vi "Main.vi"() -> ()   [LabVIEW 2023]
doc: "This Continuous Measurement sample project is based on the Queued Message Handler template.\n\nThe Event Handling Loop generates messages based on user interface actions.\n\nThe Message Handling Loop processes messages generated by the Event Handling Loop, or by other messages. There are also Acquisition and Logging message handling loop subVIs, and a chart updating loop."
uses:
  controls/UI Data.ctl
  controls/UI State.ctl
  support/Message Queue/Enqueue Message (Single).vi
  <vilib>/Utility/error.llb/Error Cluster From Error Code.vi
  <vilib>/ErrorRing/Error Ring.xnode
  Acquisition/Acquisition.lvlib
  Logging/Logging.lvlib
  support/User Event - Stop/User Event - Stop.lvlib
  support/Message Queue/Message Queue.lvlib
panel:
  out "CPU":dbl
  out "Data":u32(graph)
  in  "Start":bool
  in  "Stop":bool
  out "Status":string
  in  "Exit":bool
  # "Continuous Measurement Data Logger"
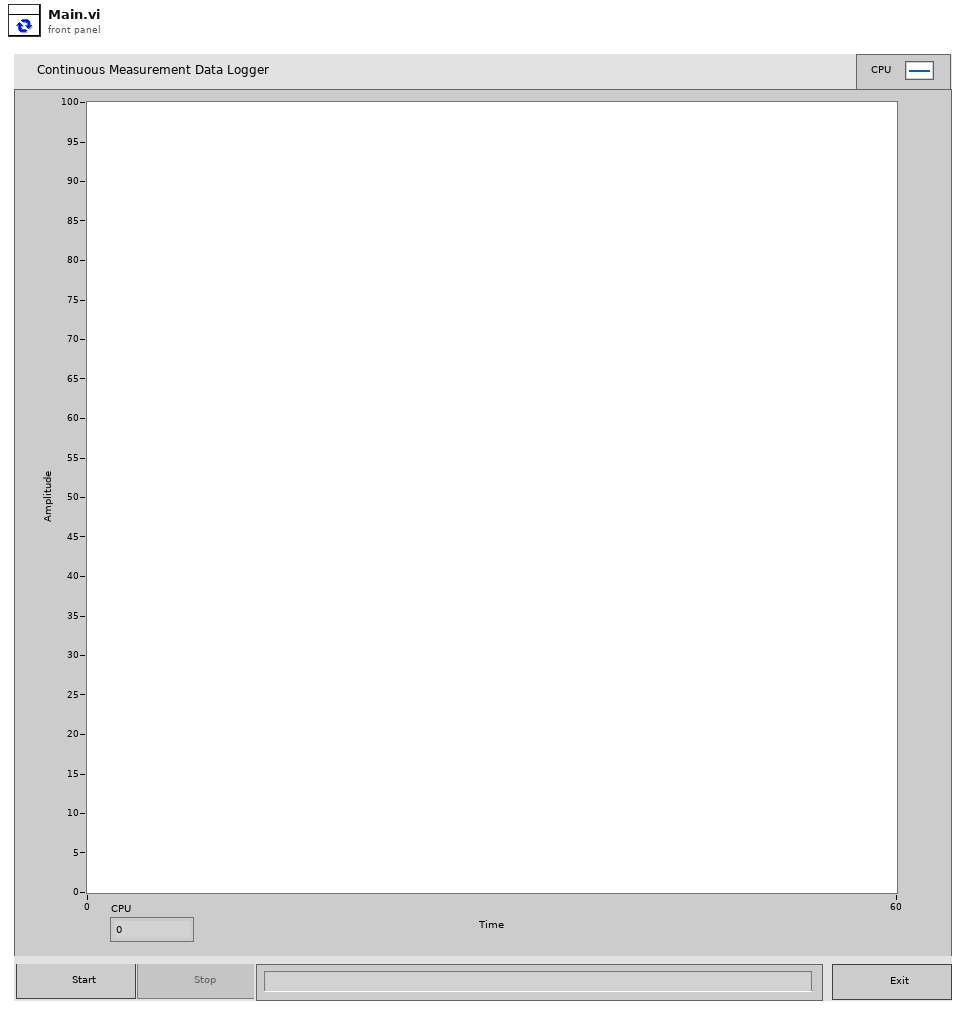
[diagram p1: front panel]
types:
  T1 = typedef "UI State.ctl" = enum16{"Idle", "Acquiring and Logging", "Waiting for Exit", "Waiting for Exit (Acq Stopped)", "Waiting for Exit (Log Stopped)", "Waiting for Stop", "Waiting for Stop (Acq Stopped)", "Waiting for Stop (Log Stopped)"}
  T2 = typedef "UI Data.ctl" = cluster{"Start Ref":refnum<vi>, "Stop Ref":refnum<vi>, "Settings Ref":refnum<vi>, "Exit Ref":refnum<vi>, "Status Ref":refnum<vi>, "Data Ref":refnum<vi>}
  T3 = typedef "Message Queue.lvlib/All Message Queues.ctl" = cluster{"UI":refnum<queue>, "Acquisition":refnum<queue>, "Logging":refnum<queue>}
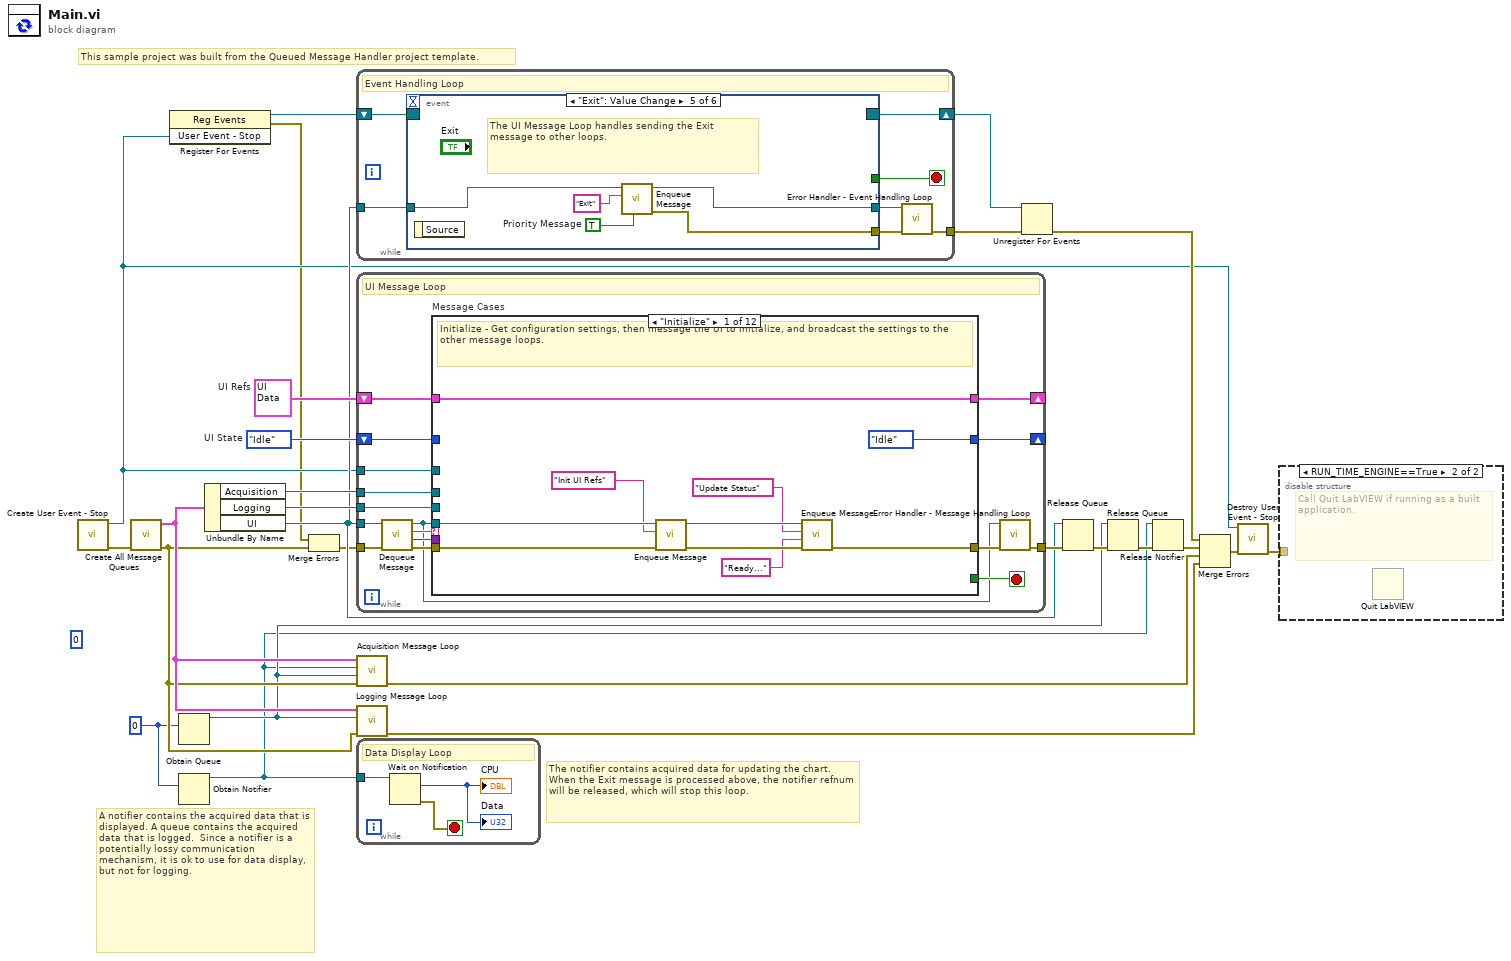
[diagram p0: block diagram]
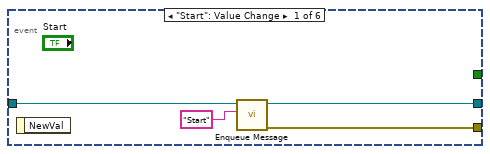
[diagram p3: hidden frame]
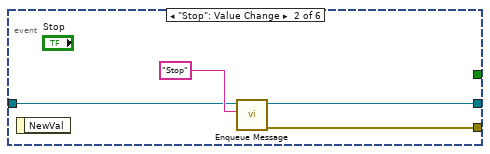
[diagram p4: hidden frame]
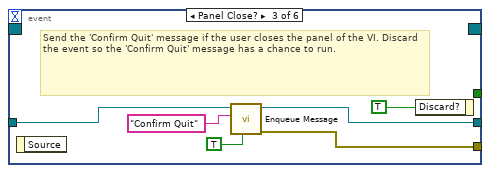
[diagram p5: hidden frame]
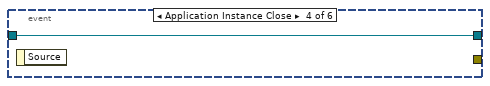
[diagram p6: hidden frame]
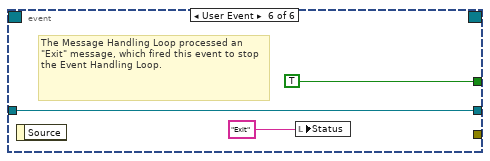
[diagram p7: hidden frame]
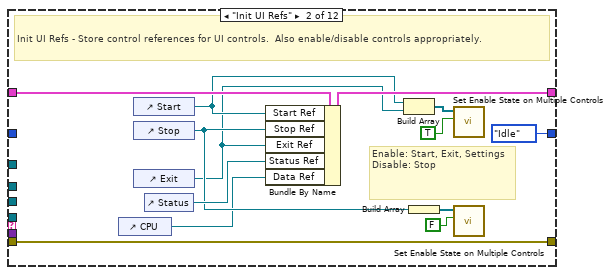
[diagram p8: hidden frame]
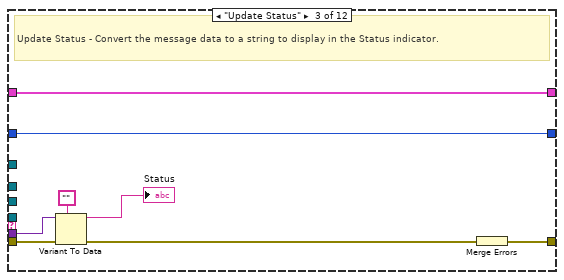
[diagram p9: hidden frame]
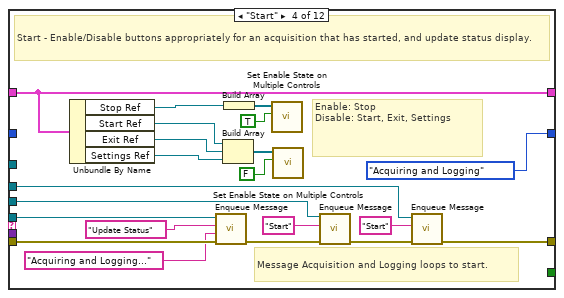
[diagram p10: hidden frame]
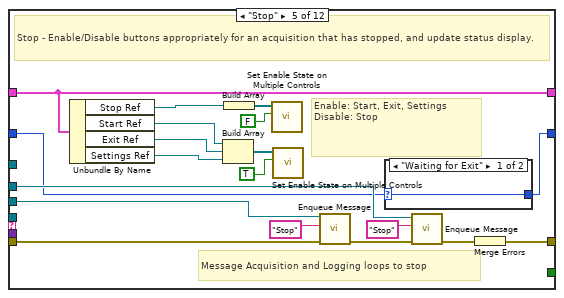
[diagram p11: hidden frame]
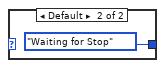
[diagram p12: hidden frame]
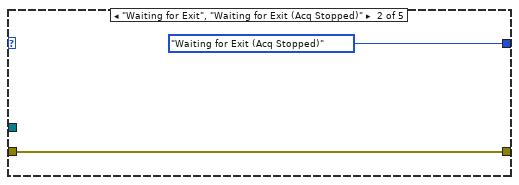
[diagram p14: hidden frame]
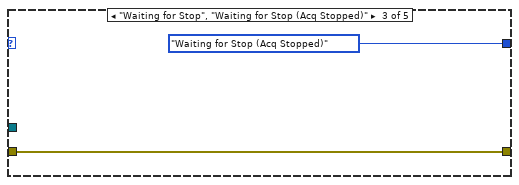
[diagram p15: hidden frame]
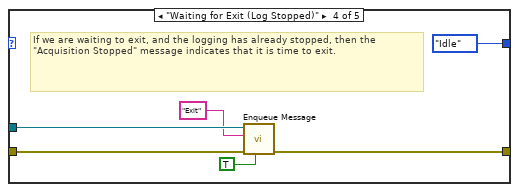
[diagram p16: hidden frame]
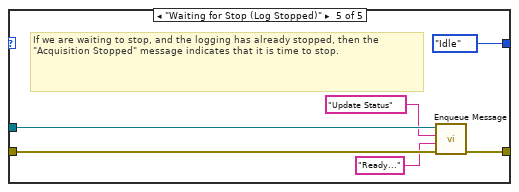
[diagram p17: hidden frame]
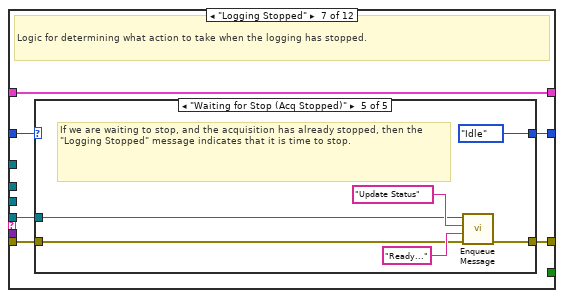
[diagram p18: hidden frame]
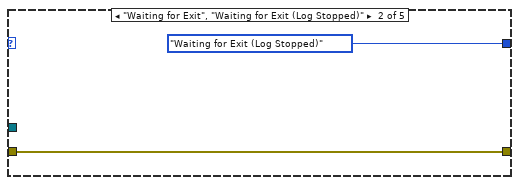
[diagram p20: hidden frame]
diagram:
  (unwired) u32 0 ("notification")
  w1 = u32 0 ("CPU load 2")
  w14 = UI_State."Idle"  # UI State
  w17 = T2 {"Start Ref"=refnum, "Stop Ref"=refnum, "Settings Ref"=refnum, "Exit Ref"=refnum, "Status Ref"=refnum, "Data Ref"=refnum}  # UI Refs
  # "This sample project was built from the Queued Message Handler project template."
  # "A notifier contains the acquired data that is displayed. A queue contains the acquired data that is logged.  Since a notifier is a potentially lossy communication mechanism, it is ok to use for data display, but not for logging."
  # "The notifier contains acquired data for updating the chart. When the Exit message is processed above, the notifier refnum will be released, which will stop this loop."
  n1 = call "Create User Event - Stop.vi"() -> ("error out"=w23:errorcluster, "User Event - Stop"=w4:refnum<user-event>)  [unwired: 10 in]
  n2 = call "Create All Message Queues.vi"("error in (no error)"=w23) -> ("error out"=w20:errorcluster, "Message Queues out"=w22:T3)  [unwired: 9 in]
  n3 = register-events(w4) -> (reference out=w5:refnum<event-registration>, error out=w2:errorcluster)  [unwired: 2 in]
  n4 = Obtain Queue(element data type=w1) -> (queue out=w7:refnum<queue>)  [unwired: 4 in, 2 out]
  n5 = Obtain Notifier(notification data type=w1) -> (notifier out=w6:refnum<notifier>)  [unwired: 3 in, 2 out]
  n6 = Unbundle By Name(w22) -> ("Acquisition"=w16:refnum<queue>, "Logging"=w15:refnum<queue>, "UI"=w12:refnum<queue>)
  n7 = Merge Errors(w2, w20) -> (w3:errorcluster)
  n8 = while {
    tunnel: w12 -> [w32]
    tunnel: [w29] -> w25
    shift-right: [w31] -> w18
    shift-left: w5 -> [w33]
    stop <- w30 stop-if-true
    # "Event Handling Loop"
    n9 = event shown="[4] \"Exit\": Value Change" {
      selector: w33 -> [_ _ _ _ _ _]
      dyn-events: [_ _ _ _ _ _] -> w31
      timeout: _ -> [_ _ _ _ _ _]
      tunnel: [_ _ _ _ _ TRUE ("Discard?")] -> w30
      tunnel: w32 -> [w37 w40 w45 w48 w50 w54]
      tunnel: [w35 w39 w43 _ w53 _] -> w28
      tunnel: [w34 w38 w44 w48 w49 w54] -> w27
      event "Start": Value Change {
        n10 = event-data() -> ()  [unwired: 1 in, 1 out]
        n11 = call-poly "Enqueue Message.vi"("Message"="Start", "Message Queue"=w37) -> ("error out"=w35:errorcluster, "dup Message Queue"=w34:refnum<queue>)  [unwired: 8 in]
      }
      event "Stop": Value Change {
        n12 = event-data() -> ()  [unwired: 1 in, 1 out]
        n13 = call-poly "Enqueue Message.vi"("Message"="Stop", "Message Queue"=w40) -> ("error out"=w39:errorcluster, "dup Message Queue"=w38:refnum<queue>)  [unwired: 8 in]
      }
      event Panel Close? {
        # "Send the 'Confirm Quit' message if the user closes the panel of the VI. Discard the event so the 'Confirm Quit' message has a chance to run."
        n14 = event-data() -> ()  [unwired: 1 in, 1 out]
        n15 = call-poly "Enqueue Message.vi"("Priority Message? (F)"=TRUE, "Message"="Confirm Quit", "Message Queue"=w45) -> ("error out"=w43:errorcluster, "dup Message Queue"=w44:refnum<queue>)  [unwired: 7 in]
        n16 = event-data("Discard?"=TRUE) -> ()  [unwired: 1 in, 1 out]
      }
      event Application Instance Close {
        n17 = event-data() -> ()  [unwired: 1 in, 1 out]
      }
      event "Exit": Value Change {
        w51 = TRUE  # Priority Message
        # "The UI Message Loop handles sending the Exit message to other loops."
        n18 = event-data() -> ()  [unwired: 1 in, 1 out]
        n19 = call-poly "Enqueue Message.vi"("Priority Message? (F)"=w51, "Message"="Exit", "Message Queue"=w50) -> ("error out"=w53:errorcluster, "dup Message Queue"=w49:refnum<queue>)  [unwired: 7 in]
      }
      event User Event {
        # "The Message Handling Loop processed an \"Exit\" message, which fired this event to stop the Event Handling Loop."
        n20 = event-data() -> ()  [unwired: 1 in, 1 out]
        n21 = local write "Status"("Exit" ("Exit String")) -> ()
      }
    }
    n22 = call "Error Handler - Event Handling Loop.vi"("error in (no error)"=w28, "Message Queue"=w27) -> ("dup error in"=w29:errorcluster)  [unwired: 8 in, 1 out]
  }
  n23 = while {
    tunnel: w12 -> [w66]
    tunnel: w4 -> [w71]
    shift-right: [w64] -> _
    shift-left: w17 -> [w65]
    tunnel: w16 -> [w63]
    tunnel: w15 -> [w62]
    shift-right: [w57] -> _
    shift-left: w14 -> [w58]
    tunnel: w3 -> [w70]
    tunnel: [w61] -> w26
    stop <- w72 stop-if-true
    # "UI Message Loop"
    n24 = call "Dequeue Message.vi"("error in (no error)"=w70, "Message Queue"=w66) -> ("error out"=w69:errorcluster, "Message Data"=w67:variant, "Message"=w68:string, "dup Message Queue"=w59:refnum<queue>)  [unwired: 6 in]
    n25 = case "Message Cases" shown="\"Initialize\"" w68 {
      selector: w68 -> [_ _ _ _ _ _ _ _ _ _ _ w249]
      tunnel: w59 -> [w76 _ _ w124 _ w148 w172 _ w205 _ _ _]
      tunnel: w69 -> [w75 w95 w102 w123 w142 w149 w173 w194 w204 w232 w247 _]
      tunnel: [w80 w95 w103 w107 w143 w146 w170 w197 w203 w241 w246 w248] -> w60
      tunnel: [_ _ _ _ _ _ _ _ _ TRUE _ _] -> w72
      tunnel: w67 -> [_ _ w101 _ _ _ _ w198 _ w230 _ _]
      tunnel: w71 -> [_ _ _ _ _ _ _ _ _ w242 _ _]
      tunnel: w65 -> [w77 w94 w97 w120 w141 w151 w175 w201 w207 w240 w245 w251]
      tunnel: [w77 w92 w97 w120 w141 w151 w175 w201 w207 w240 w245 w251] -> w64
      tunnel: w63 -> [_ _ _ w106 w128 _ _ _ _ w239 _ _]
      tunnel: w62 -> [_ _ _ w109 w131 _ _ _ _ w238 _ _]
      tunnel: w58 -> [_ _ w96 _ w125 w150 w174 w196 w206 _ w244 w250]
      tunnel: [UI_State."Idle" ("UI State") UI_State."Idle" ("UI State") w96 UI_State."Acquiring and Logging" ("UI State") w126 w147 w171 w196 w202 UI_State."Idle" ("UI State") w244 w250] -> w57
      frame "Initialize" {
        # "Initialize - Get configuration settings, then message the UI to initialize, and broadcast the settings to the other message loops."
        n26 = call-poly "Enqueue Message.vi"("error in (no error)"=w75, "Message"="Init UI Refs", "Message Queue"=w76) -> ("error out"=w82:errorcluster, "dup Message Queue"=w81:refnum<queue>)  [unwired: 7 in]
        n27 = call-poly "Enqueue Message.vi"("error in (no error)"=w82, "Message Data"="Ready..." ("Ready..."), "Message"="Update Status", "Message Queue"=w81) -> ("error out"=w80:errorcluster)  [unwired: 6 in, 1 out]
      }
      frame "Init UI Refs" {
        # "Enable: Start, Exit, Settings\nDisable: Stop"
        # "Init UI Refs - Store control references for UI controls.  Also enable/disable controls appropriately."
        n28 = control-ref of="CPU"() -> (w83:refnum<vi>)
        n29 = control-ref of="Start"() -> (w86:refnum<vi>)
        n30 = control-ref of="Stop"() -> (w87:refnum<vi>)
        n31 = control-ref of="Exit"() -> (w84:refnum<vi>)
        n32 = control-ref of="Status"() -> (w93:refnum<vi>)
        n33 = Bundle By Name(cluster=w94, "Start Ref"=w86, "Stop Ref"=w87, "Exit Ref"=w84, "Status Ref"=w93, "Data Ref"=w83) -> (w92:T2)
        n34 = Build Array(w86, w84) -> (w90:refnum<vi>[])
        n35 = Build Array(w87) -> (w89:refnum<vi>[])
        n36 = call "Set Enable State on Multiple Controls.vi"("Enable?"=TRUE, "Controls"=w90) -> ()  [unwired: 10 in]
        n37 = call "Set Enable State on Multiple Controls.vi"("Enable?"=FALSE, "Controls"=w89) -> ()  [unwired: 10 in]
      }
      frame "Update Status" {
        # "Update Status - Convert the message data to a string to display in the Status indicator."
        n38 = Variant To Data(error in=w102, type="", Variant=w101) -> (data=→"Status":string, error out=w99:errorcluster)
        n39 = Merge Errors(w99) -> (w103:errorcluster)
      }
      frame "Start" {
        # "Message Acquisition and Logging loops to start."
        # "Enable: Stop\nDisable: Start, Exit, Settings"
        # "Start - Enable/Disable buttons appropriately for an acquisition that has started, and update status display."
        n40 = Unbundle By Name(w120) -> ("Stop Ref"=w115:refnum<vi>, "Start Ref"=w114:refnum<vi>, "Exit Ref"=w113:refnum<vi>, "Settings Ref"=w112:refnum<vi>)
        n41 = call-poly "Enqueue Message.vi"("error in (no error)"=w123, "Message Data"="Acquiring and Logging..." ("Acquiring and Logging..."), "Message"="Update Status", "Message Queue"=w124) -> ("error out"=w111:errorcluster)  [unwired: 6 in, 1 out]
        n42 = Build Array(w114, w113, w112) -> (w118:refnum<vi>[])
        n43 = Build Array(w115) -> (w117:refnum<vi>[])
        n44 = call "Set Enable State on Multiple Controls.vi"("Enable?"=TRUE, "Controls"=w117) -> ()  [unwired: 10 in]
        n45 = call "Set Enable State on Multiple Controls.vi"("Enable?"=FALSE, "Controls"=w118) -> ()  [unwired: 10 in]
        n46 = call-poly "Enqueue Message.vi"("error in (no error)"=w111, "Message"="Start", "Message Queue"=w109) -> ("error out"=w108:errorcluster)  [unwired: 7 in, 1 out]
        n47 = call-poly "Enqueue Message.vi"("error in (no error)"=w108, "Message"="Start", "Message Queue"=w106) -> ("error out"=w107:errorcluster)  [unwired: 7 in, 1 out]
      }
      frame "Stop" {
        # "Message Acquisition and Logging loops to stop"
        # "Enable: Start, Exit, Settings\nDisable: Stop"
        # "Stop - Enable/Disable buttons appropriately for an acquisition that has stopped, and update status display."
        n48 = Unbundle By Name(w141) -> ("Stop Ref"=w136:refnum<vi>, "Start Ref"=w135:refnum<vi>, "Exit Ref"=w134:refnum<vi>, "Settings Ref"=w133:refnum<vi>)
        n49 = Build Array(w135, w134, w133) -> (w139:refnum<vi>[])
        n50 = Build Array(w136) -> (w138:refnum<vi>[])
        n51 = call "Set Enable State on Multiple Controls.vi"("Enable?"=FALSE, "Controls"=w138) -> ()  [unwired: 10 in]
        n52 = call "Set Enable State on Multiple Controls.vi"("Enable?"=TRUE, "Controls"=w139) -> ()  [unwired: 10 in]
        n53 = call-poly "Enqueue Message.vi"("error in (no error)"=w142, "Message"="Stop", "Message Queue"=w131) -> ("error out"=w130:errorcluster)  [unwired: 7 in, 1 out]
        n54 = case shown="\"Waiting for Exit\"" w125 {
          selector: w125 -> [w144 _]
          tunnel: [w144 UI_State."Waiting for Stop" ("UI State")] -> w126
          frame "Waiting for Exit" {
          }
          frame Default {
          }
        }
        n55 = call-poly "Enqueue Message.vi"("error in (no error)"=w130, "Message"="Stop", "Message Queue"=w128) -> ("error out"=w129:errorcluster)  [unwired: 7 in, 1 out]
        n56 = Merge Errors(w129) -> (w143:errorcluster)
      }
      frame "Acquisition Stopped" {
        # "Logic for determining what action to take when the acquisition has stopped."
        n57 = case shown="Default" w150 {
          selector: w150 -> [w153 _ _ _ _]
          tunnel: w149 -> [w152 w155 w157 w163 w169]
          tunnel: w148 -> [_ _ _ w161 w166]
          tunnel: [w153 UI_State."Waiting for Exit (Acq Stopped)" ("UI State") UI_State."Waiting for Stop (Acq Stopped)" ("UI State") UI_State."Idle" ("UI State") UI_State."Idle" ("UI State")] -> w147
          tunnel: [w152 w155 w157 w162 w167] -> w146
          frame Default {
          }
          frame "Waiting for Exit", "Waiting for Exit (Acq Stopped)" {
          }
          frame "Waiting for Stop", "Waiting for Stop (Acq Stopped)" {
          }
          frame "Waiting for Exit (Log Stopped)" {
            # "If we are waiting to exit, and the logging has already stopped, then the \"Acquisition Stopped\" message indicates that it is time to exit."
            n58 = call-poly "Enqueue Message.vi"("Priority Message? (F)"=TRUE, "error in (no error)"=w163, "Message"="Exit", "Message Queue"=w161) -> ("error out"=w162:errorcluster)  [unwired: 6 in, 1 out]
          }
          frame "Waiting for Stop (Log Stopped)" {
            # "If we are waiting to stop, and the logging has already stopped, then the \"Acquisition Stopped\" message indicates that it is time to stop."
            n59 = call-poly "Enqueue Message.vi"("error in (no error)"=w169, "Message Data"="Ready..." ("Ready..."), "Message"="Update Status", "Message Queue"=w166) -> ("error out"=w167:errorcluster)  [unwired: 6 in, 1 out]
          }
        }
      }
      frame "Logging Stopped" {
        # "Logic for determining what action to take when the logging has stopped."
        n60 = case shown="\"Waiting for Stop (Acq Stopped)\"" w174 {
          selector: w174 -> [w177 _ _ _ _]
          tunnel: w173 -> [w176 w179 w181 w187 w190]
          tunnel: w172 -> [_ _ _ w185 w189]
          tunnel: [w177 UI_State."Waiting for Exit (Log Stopped)" ("UI State") UI_State."Waiting for Stop (Log Stopped)" ("UI State") UI_State."Idle" ("UI State") UI_State."Idle" ("UI State")] -> w171
          tunnel: [w176 w179 w181 w186 w188] -> w170
          frame Default {
          }
          frame "Waiting for Exit", "Waiting for Exit (Log Stopped)" {
          }
          frame "Waiting for Stop", "Waiting for Stop (Log Stopped)" {
          }
          frame "Waiting for Exit (Acq Stopped)" {
            # "If we are waiting to exit, and the acquisition has already stopped, then the \"Logging Stopped\" message indicates that it is time to exit."
            n61 = call-poly "Enqueue Message.vi"("Priority Message? (F)"=TRUE, "error in (no error)"=w187, "Message"="Exit", "Message Queue"=w185) -> ("error out"=w186:errorcluster)  [unwired: 6 in, 1 out]
          }
          frame "Waiting for Stop (Acq Stopped)" {
            # "If we are waiting to stop, and the acquisition has already stopped, then the \"Logging Stopped\" message indicates that it is time to stop."
            n62 = call-poly "Enqueue Message.vi"("error in (no error)"=w190, "Message Data"="Ready..." ("Ready..."), "Message"="Update Status", "Message Queue"=w189) -> ("error out"=w188:errorcluster)  [unwired: 6 in, 1 out]
          }
        }
      }
      frame "Error" {
        # "Error - Display an error dialog. This message is sent by the \"Error Handler\" VIs at the end of other loops in this application."
        n63 = Variant To Data(error in=w194, type=errorcluster {"status"=FALSE, "code"=0, "source"=""} ("error constant"), Variant=w198) -> (data=w195:errorcluster, error out=w199:errorcluster)
        n64 = call <vilib>:"Simple Error Handler.vi"("error in (no error)"=w195) -> ()  [unwired: 4 in, 5 out]
        n65 = Merge Errors(w199) -> (w197:errorcluster)
      }
      frame "Confirm Quit" {
        # "Confirm Quit - Message that can confirm whether or not the user wants to exit the application."
        n66 = case shown="\"Acquiring and Logging\"" w206 {
          tunnel: w205 -> [w213 w217]
          tunnel: w204 -> [w212 w216]
          tunnel: [w211 w215] -> w203
          tunnel: [UI_State."Idle" ("UI State") w214] -> w202
          frame Default {
            # "If 'Confirm Quit' comes in while the system is idle, there is no need for a confirmation message."
            n67 = call-poly "Enqueue Message.vi"("Priority Message? (F)"=TRUE, "error in (no error)"=w212, "Message"="Exit", "Message Queue"=w213) -> ("error out"=w211:errorcluster)  [unwired: 6 in, 1 out]
          }
          frame "Acquiring and Logging" {
            n68 = Two Button Dialog(message="Are you sure you want to quit while the acquisition is running?" ("Confirm Quit Message"), 1:"No" ("No"), 2:"Yes" ("Yes")) -> (T button?=w218:bool)
            n69 = case shown="True" w218 {
              tunnel: w217 -> [_ w227]
              tunnel: w216 -> [w223 w228]
              tunnel: [w223 w226] -> w215
              tunnel: [UI_State."Acquiring and Logging" ("UI State") UI_State."Waiting for Exit" ("UI State")] -> w214
              frame False {
                # "User did not want to quit."
              }
              frame True {
                n70 = call-poly "Enqueue Message.vi"("error in (no error)"=w228, "Message"="Stop", "Message Queue"=w227) -> ("error out"=w226:errorcluster)  [unwired: 7 in, 1 out]
              }
            }
          }
        }
      }
      frame "Exit" {
        w234 = TRUE ("Priority Message? (F)")
        w235 = "Exit" ("Message")
        # "Popup an error dialog if 'Exit' was called as a result of an error."
        # "Stop the VI"
        # "Exit - Send Exit messages to the Acquisition and Logging loops, and fire the user event to stop the Event Handling Loop."
        n71 = Variant To Data(type=errorcluster {"status"=FALSE, "code"=0, "source"=""} ("error constant"), Variant=w230) -> (data=w229:errorcluster)  [unwired: 1 in, 1 out]
        n72 = call <vilib>:"Simple Error Handler.vi"("error in (no error)"=w229) -> ()  [unwired: 4 in, 5 out]
        n73 = call-poly "Enqueue Message.vi"("Priority Message? (F)"=w234, "error in (no error)"=w232, "Message"=w235, "Message Queue"=w239) -> ("error out"=w236:errorcluster)  [unwired: 6 in, 1 out]
        n74 = call-poly "Enqueue Message.vi"("Priority Message? (F)"=w234, "error in (no error)"=w236, "Message"=w235, "Message Queue"=w238) -> ("error out"=w233:errorcluster)  [unwired: 6 in, 1 out]
        n75 = call "Fire User Event - Stop.vi"("error in (no error)"=w233, "User Event - Stop"=w242) -> ("error out"=w241:errorcluster)  [unwired: 9 in]
      }
      frame "---Copy This Frame---" {
        # "Duplicate this frame when creating new messages.  Change this comment in the duplicated frame to describe this message."
        n76 = Merge Errors(w247) -> (w246:errorcluster)
      }
      frame Default {
        # "'Default' case only runs if there is a message that isn't defined in any of the other cases.  Output a programming error."
        n77 = xnode "Error Ring"("parameter 0"=w249) -> ("error out"=w248:errorcluster)
      }
    }
    n78 = call "Error Handler - Message Handling Loop.vi"("error in (no error)"=w60, "Message Queue"=w59) -> ("dup error in"=w61:errorcluster)  [unwired: 8 in, 1 out]
  }
  n79 = call "Acquisition Message Loop.vi"("error in (no error)"=w20, "Data Queue"=w7, "Data Notifier"=w6, "Message Queues"=w22) -> ("error out"=w24:errorcluster)  [unwired: 7 in]
  n80 = call "Logging Message Loop.vi"("error in (no error)"=w20, "Data Queue"=w7, "Message Queues"=w22) -> ("error out"=w21:errorcluster)  [unwired: 8 in]
  n81 = while "Data Display Loop" {
    tunnel: w6 -> [w261]
    stop <- w260 stop-if-true
    # "Data Display Loop"
    n82 = Wait on Notification(notifier=w261) -> (notification=→"Data" →"CPU":u32, error out=w260:errorcluster)  [unwired: 3 in, 2 out]
  }
  n83 = Unregister For Events(event registration refnum=w18, error in=w25) -> (error out=w19:errorcluster)
  n84 = Release Queue(queue=w12, error in (no error)=w26) -> (error out=w10:errorcluster)  [unwired: 1 in, 2 out]
  n85 = Release Queue(queue=w7, error in (no error)=w10) -> (error out=w9:errorcluster)  [unwired: 1 in, 2 out]
  n86 = Release Notifier(notifier=w6, error in (no error)=w9) -> (error out=w8:errorcluster)  [unwired: 1 in, 2 out]
  n87 = Merge Errors(w19, w8, w24, w21) -> (w13:errorcluster)
  n88 = call "Destroy User Event - Stop.vi"("error in (no error)"=w13, "User Event - Stop"=w4) -> ("error out"=w11:errorcluster)  [unwired: 9 in]
  n89 = disable-structure shown="RUN_TIME_ENGINE==True" {
    disable-tunnel: w11 -> [_ _]
    frame condition #0 (active) {
    }
    frame condition #1 {
      # "Call Quit LabVIEW if running as a built application."
      n90 = Quit LabVIEW() -> ()  [unwired: 1 in]
    }
  }
